vi "DiffDriveTrainSim_GetLeftPositionMeters.vi"(11 "DiffDriveTrainSim":T1 {"m_Motor"."Jr_KgM2" format="%13.5p"; "m_Motor"."L_H" format="%13.5p"; "m_Motor"."Kt_NMPerAmp" format="%13.5p"; "m_Motor"."KvINV_RadPerSecPerVolt" format="%13.5p"; "m_Motor"."R_Ohms" format="%13.5p"; "m_Motor"."FreeSpeed_RadPerSec" format="%13.5p"; "m_Motor"."FreeCurrent_Amps" format="%13.5p"; "m_Motor"."StallCurrent_Amps" format="%13.5p"; "m_Motor"."StallTorque_NM" format="%13.5p"; "m_Motor"."nominalVoltage_Volts" format="%13.5p"}) -> (3 "LeftPosition_Meters":dbl)   [LabVIEW 2019, in "Trajectory_Library.lvlib"]
doc: "Get the left encoder position in meters.\n \nInputs:\n - DiffDriveTraimSim -- Data cluster\n\nOutputs:\n - LeftPosition_Meters -- The encoder position."
uses:
  Trajectory_Library.lvlib
  DIFF_DRIVE_TRAIN_SIM.ctl
  LINEAR_SYSTEM.ctl
  <vilib>/Analysis/Matrix/Datatypes/RealMatrix.ctl
  DCMOTOR.CTL
  <vilib>/Analysis/Matrix/NI_Matrix.lvlib
panel:
  # "<States, 1>"
  # "<Outputs, 1>"
  # "<Inputs, 1>"
  # "<Outputs, 1>"
  # "<States,States>"
  # "<States,Inputs>"
  # "<Outputs,States>"
  # "<Outputs,Inputs>"
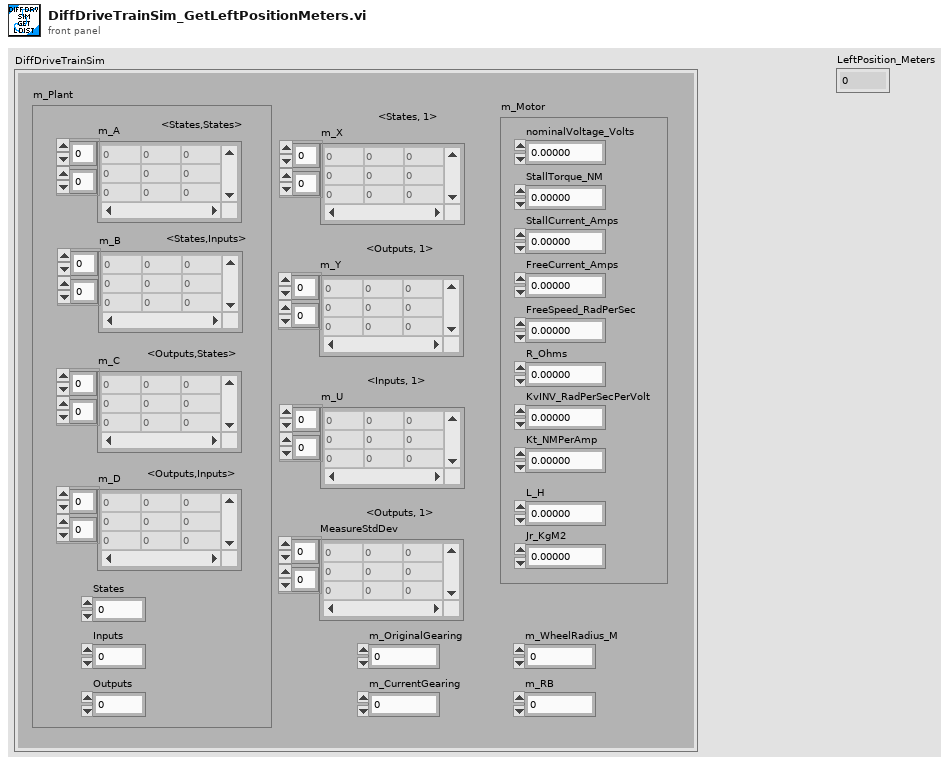
[diagram p1: front panel]
types:
  T1 = typedef "Trajectory_Library.lvlib/DIFF_DRIVE_TRAIN_SIM.ctl" = cluster{"m_Plant":T2, "m_X":T3, "m_Y":T3, "m_U":T3, "MeasureStdDev":T3, "m_Motor":T4, "m_OriginalGearing":dbl, "m_CurrentGearing":dbl, "m_WheelRadius_M":dbl, "m_RB":dbl}
  T2 = typedef "Trajectory_Library.lvlib/LINEAR_SYSTEM.ctl" = cluster{"m_A":T3, "m_B":T3, "m_C":T3, "m_D":T3, "States":i32, "Inputs":i32, "Outputs":i32}
  T3 = typedef "NI_Matrix.lvlib/RealMatrix.ctl" = dbl[][]
  T4 = typedef "Trajectory_Library.lvlib/DCMOTOR.CTL" = cluster{"nominalVoltage_Volts":dbl, "StallTorque_NM":dbl, "StallCurrent_Amps":dbl, "FreeCurrent_Amps":dbl, "FreeSpeed_RadPerSec":dbl, "R_Ohms":dbl, "KvINV_RadPerSecPerVolt":dbl, "Kt_NMPerAmp":dbl, "L_H":dbl, "Jr_KgM2":dbl}
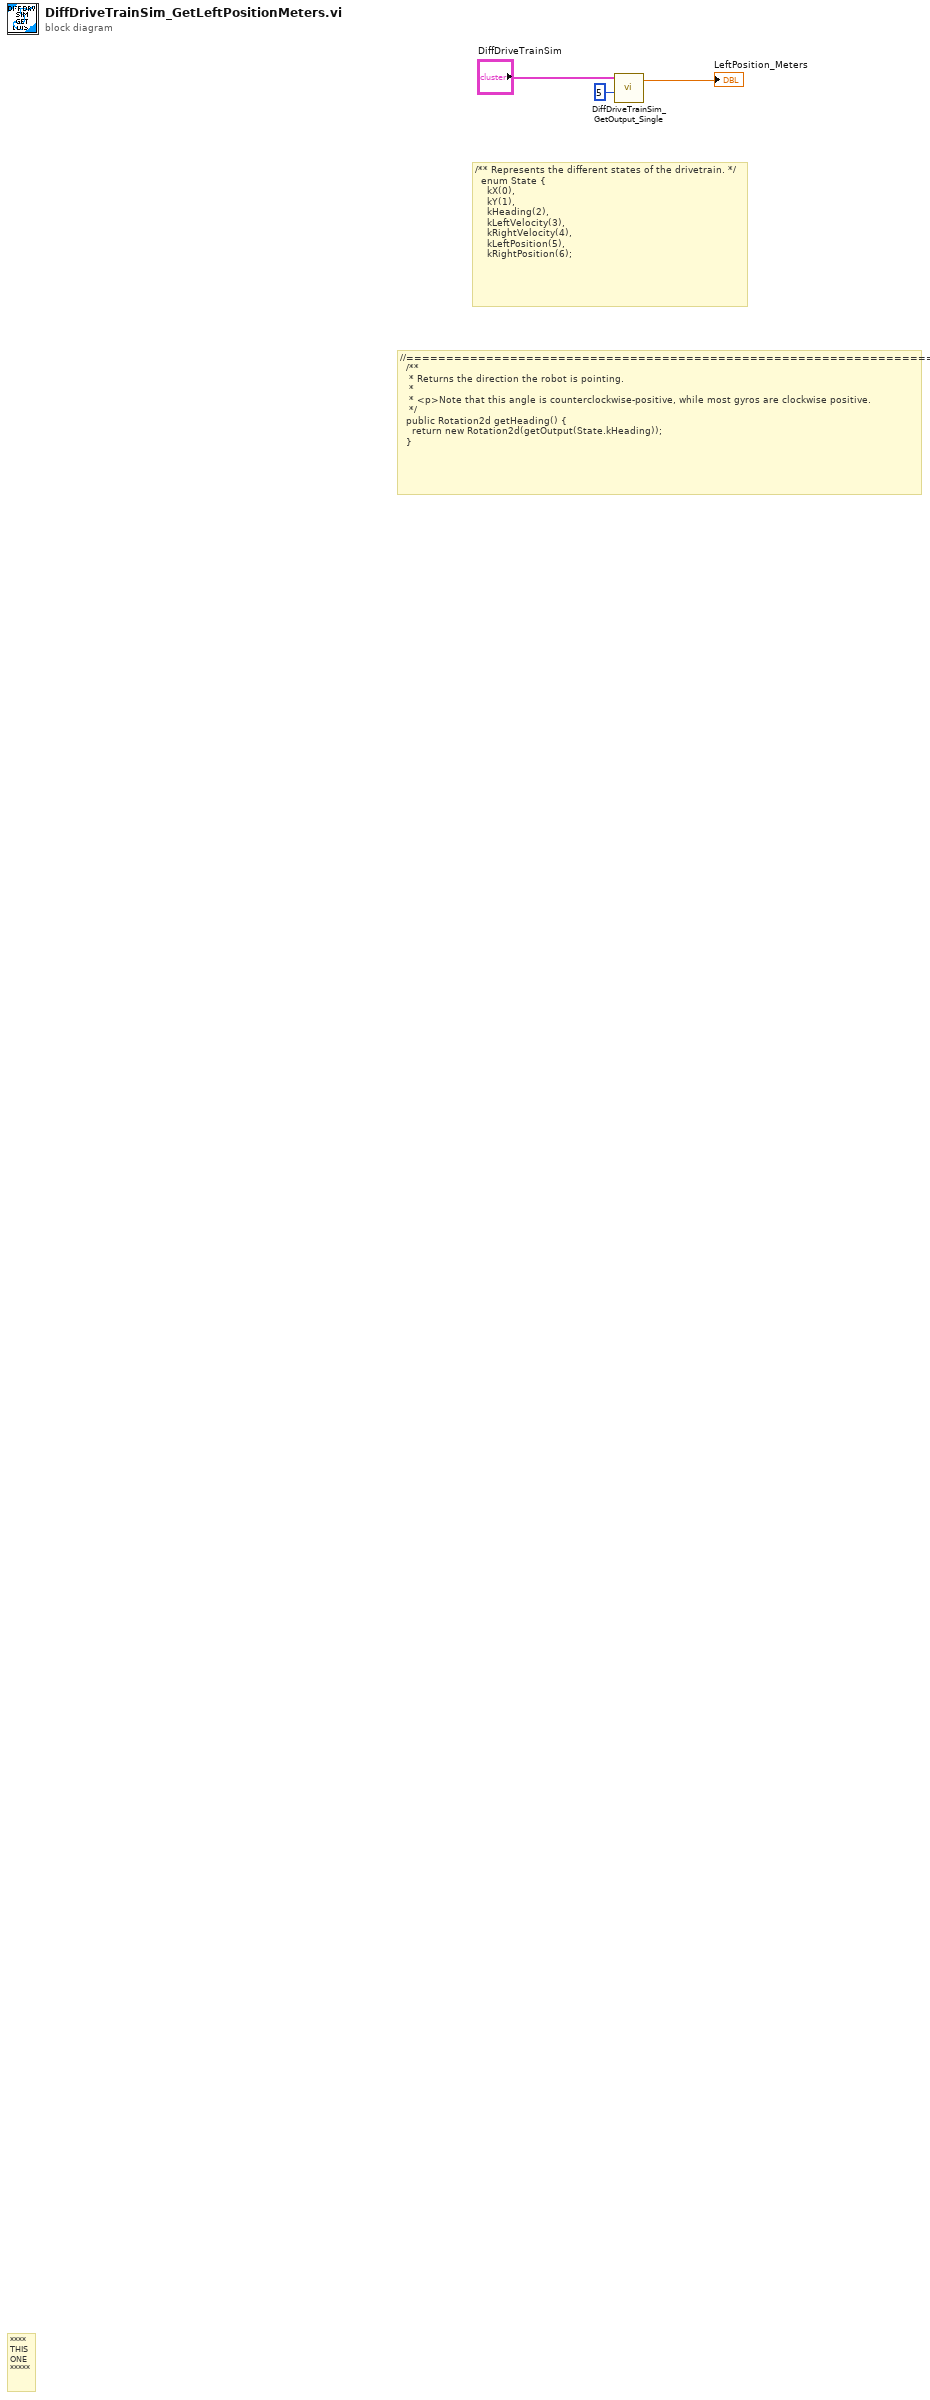
[diagram p0: block diagram]
diagram:
  # "/** Represents the different states of the drivetrain. */\n  enum State {\n    kX(0),\n    kY(1),\n    kHeading(2),\n    kLeftVelocity(3),\n    kRightVelocity(4),\n    kLeftPosition(5),\n    kRightPosition(6);"
  # "//===================================================================\n  /**\n   * Returns the direction the robot is pointing.\n   *\n   * <p>Note that this angle is counterclockwise-positive, while most gyros are clockwise positive.\n   */\n  public Rotation2d getHeading() {\n    return new Rotation2d(getOutput(State.kHeading));\n  }"
  # "****\nTHIS\nONE\n*****"
  n1 = call "DiffDriveTrainSim_GetOutput_Single.vi"("Row"=5, "DiffDriveTrainSim"="DiffDriveTrainSim") -> ("Output"=→"LeftPosition_Meters":dbl)  [unwired: 9 in]
